vi "WLAN_RSMA_FrameBuild - 16QAM.vi"(7 "Alpha":dbl min=0.0 max=1.0 step=0.05 format="%#_13g", 8 "error in (no error)":errorcluster, 9 "data in 2":i8[](array[numeric]) caption="input bit stream", 10 "Modulation parameter":T2, 11 "data in":i8[](array[numeric]) caption="input bit stream") -> (0 "error out":errorcluster, 3 "output array":cdb[](array[numeric]))   [LabVIEW 2022 SP3]
panel:
  in  "Modulation type":T1(ring)=enum."16QAM"
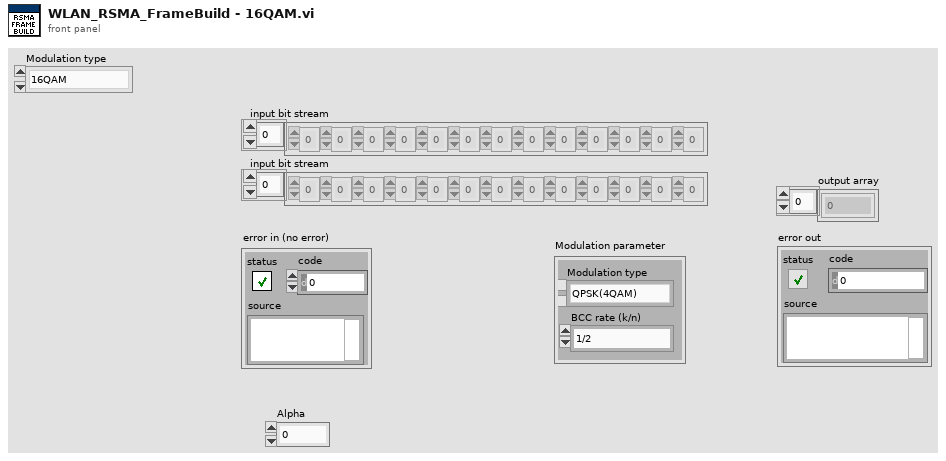
[diagram p1: front panel]
types:
  T1 = enum16{"QPSK(4QAM)", "64QAM", "16QAM", "BPSK", "BPSK Vertical"}
  T2 = cluster{"Modulation type":enum16{"QPSK(4QAM)", "64QAM", "16QAM", "BPSK"}, "BCC rate (k/n)":enum16{"1/2", "2/3", "3/4"}}
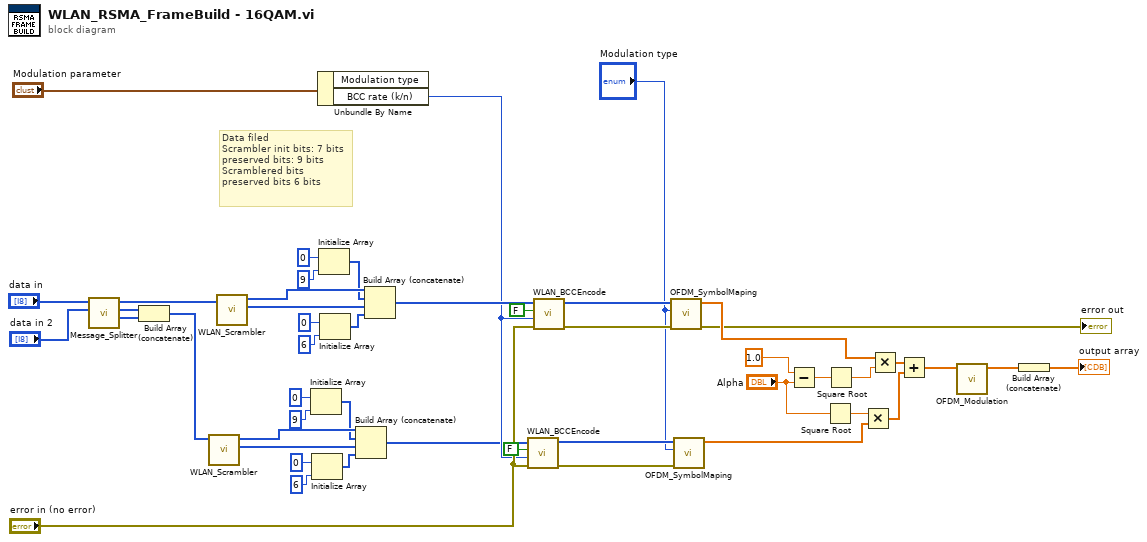
[diagram p0: block diagram]
diagram:
  # "Data filed\nScrambler init bits: 7 bits\npreserved bits: 9 bits\nScramblered bits\npreserved bits 6 bits"
  n1 = call "Message_Splitter.vi"("W2"="data in 2", "W1"="data in") -> ("Wp2"=w4:u8[], "Wp1"=w5:u8[], "Wc"=w3:u8[])  [unwired: 7 in]
  n2 = Build Array (concatenate)(w5, w4) -> (w2:u8[])
  n3 = call "WLAN_Scrambler.vi"("input bit stream"=w2) -> ("scrambled bits"=w23:i8[], "scrambler initial bit"=w27:i8[])  [unwired: 9 in]
  n4 = call "WLAN_Scrambler.vi"("input bit stream"=w3) -> ("scrambled bits"=w19:i8[], "scrambler initial bit"=w34:i8[])  [unwired: 9 in]
  n5 = Initialize Array(i8 0 ("element"), 9 ("dimension size")) -> (w26:i8[])
  n6 = Initialize Array(i8 0 ("element"), 6 ("dimension size")) -> (w20:i8[])
  n7 = Unbundle By Name("Modulation parameter") -> ("BCC rate (k/n)"=w42:enum16{"1/2", "2/3", "3/4"})  [unwired: 1 out]
  n8 = Initialize Array(i8 0 ("element"), 9 ("dimension size")) -> (w33:i8[])
  n9 = Initialize Array(i8 0 ("element"), 6 ("dimension size")) -> (w28:i8[])
  n10 = Build Array (concatenate)(w27, w26, w23, w20) -> (w39:i8[])
  n11 = Build Array (concatenate)(w34, w33, w19, w28) -> (w47:i8[])
  n12 = call "WLAN_BCCEncode.vi"("error in (no error)"="error in (no error)", "BCC rate (k/n)"=w42, "need add zeros?"=FALSE, "input bit stream"=w39) -> ("error out"=w37:errorcluster, "output bit stream 3"=w38:i8[])  [unwired: 6 in]
  n13 = call "WLAN_BCCEncode.vi"("error in (no error)"="error in (no error)", "BCC rate (k/n)"=w42, "need add zeros?"=FALSE, "input bit stream"=w47) -> ("error out"=w45:errorcluster, "output bit stream 3"=w44:i8[])  [unwired: 6 in]
  n14 = call "OFDM_SymbolMaping.vi"("error in (no error)"=w45, "Modulation type"="Modulation type", "input bit stream"=w44) -> ("error out"=→"error out":errorcluster, "symbols"=w41:cdb[])  [unwired: 7 in]
  n15 = call "OFDM_SymbolMaping.vi"("error in (no error)"=w37, "Modulation type"="Modulation type", "input bit stream"=w38) -> ("symbols"=w36:cdb[])  [unwired: 7 in, 1 out]
  n16 = Subtract(x=1.0, y="Alpha") -> (x-y=w11:dbl)
  n17 = Square Root(x="Alpha") -> (sqrt(x)=w15:dbl)
  n18 = Square Root(x=w11) -> (sqrt(x)=w13:dbl)
  n19 = Multiply(x=w15, y=w36) -> (x*y=w16:cdb[])
  n20 = Multiply(x=w41, y=w13) -> (x*y=w14:cdb[])
  n21 = Add(x=w14, y=w16) -> (x+y=w9:cdb[])
  n22 = call "OFDM_Modulation.vi"("Input sequence"=w9) -> ("Output sequence"=w8:cdb[])  [unwired: 10 in]
  n23 = Build Array (concatenate)(w8) -> (→"output array":cdb[])
